vi "GUI_TRA_v1.0.0.vi"() -> ()   [LabVIEW 2011]
uses:
  Device Driver/TRAServer/HomingType_TypDef.ctl
  Device Driver/TRAServer/StatusTRA_TypDef.ctl
  Device Driver/shared/OnOffTypeDef.ctl
  <vilib>/Utility/file.llb/Write To Spreadsheet File (string).vi
  <vilib>/Utility/file.llb/Write To Spreadsheet File (DBL).vi
  Device Driver/TRAServer/TRAServer.lvclass
panel:
  in  "Multicolumn Listbox 2":refnum<vi>
  in  "Main Tap 2":refnum<vi>
  out "all pos array":refnum<vi>[][](array[refnum])
  out "all status array":refnum<vi>[][](array[refnum])
  out "indecator ref array 2":refnum<vi>[](array[refnum])
  out "indecator ref array":refnum<vi>[](array[refnum])
  in  "time to wait (TCP) 2":i32=10
  in  "plot":bool=TRUE
  out "ratio(h)":bool
  out "fixsize":bool
  out "error (h)":bool
  out "Device Name (h)":string="StagingTRA1"
  in  "Main Tap":T1(tab)
  in  "stepSize":dbl
  in  "Status":T2=enum."DISABLE" caption="Status Y"
  in  "Up":bool
  in  "Down":bool
  in  "Right":bool
  in  "Left":bool
  in  "Status":T2=enum."DISABLE" caption="Status X"
  in  "Position":dbl=2.54999 caption="X"
  in  "Position":dbl=3.05 caption="Y"
  in  "Mirror":T3(ring)
  in  "backlash":dbl
  in  "backlash":dbl
  in  "device status":string
  in  "Home 3":bool=TRUE
  in  "Home 2":bool=TRUE
  out "Status.Axis 6":T2=enum."DISABLE" caption="Status X"
  out "Status.Axis 5":T2=enum."DISABLE" caption="Status X"
  out "Status.Axis 4":T2=enum."DISABLE" caption="Status X"
  out "Status.Axis 3":T2=enum."DISABLE" caption="Status X"
  out "Status.Axis 2":T2=enum."DISABLE" caption="Status X"
  out "Status.Axis 1":T2=enum."DISABLE" caption="Status X"
  out "Status.Axis 1":T2=enum."DISABLE" caption="Status X"
  out "Status.Axis 2":T2=enum."DISABLE" caption="Status X"
  out "Status.Axis 3":T2=enum."DISABLE" caption="Status X"
  out "Status.Axis 4":T2=enum."DISABLE" caption="Status X"
  out "Status.Axis 5":T2=enum."DISABLE" caption="Status X"
  out "Status.Axis 6":T2=enum."DISABLE" caption="Status X"
  out "Status.Axis 7":T2=enum."DISABLE" caption="Status X"
  out "Status.Axis 8":T2=enum."DISABLE" caption="Status X"
  out "Status.Axis 9":T2=enum."DISABLE" caption="Status X"
  out "Status.Axis 10":T2=enum."DISABLE" caption="Status X"
  out "Status.Axis 11":T2=enum."DISABLE" caption="Status X"
  out "Status.Axis 12":T2=enum."DISABLE" caption="Status X"
  in  "Home 1":bool=TRUE
  in  "Path":path
  in  "Save":bool
  in  "Multicolumn Listbox":i32(listbox)
  in  "Position.Axis 1":dbl=3.05 caption="X"
  in  "Position.Axis 2":dbl=3.05 caption="Y"
  in  "Position.Axis 4":dbl=3.05 caption="X"
  in  "Position.Axis 3":dbl=3.05 caption="Y"
  in  "Position.Axis 6":dbl=3.05 caption="X"
  in  "Position.Axis 5":dbl=3.05 caption="Y"
  in  "Position.Axis 18":dbl=3.05 caption="X"
  in  "Position.Axis 17":dbl=3.05 caption="Y"
  in  "Position.Axis 16":dbl=3.05 caption="X"
  in  "Position.Axis 15":dbl=3.05 caption="Y"
  in  "Position.Axis 14":dbl=3.05 caption="X"
  in  "Position.Axis 13":dbl=3.05 caption="Y"
  in  "Position.Axis 12":dbl=3.05 caption="X"
  in  "Position.Axis 11":dbl=3.05 caption="Y"
  in  "Position.Axis 10":dbl=3.05 caption="X"
  in  "Position.Axis 9":dbl=3.05 caption="Y"
  in  "Position.Axis 8":dbl=3.05 caption="Y"
  in  "Position.Axis 7":dbl=3.05 caption="X"
  in  "take images":bool
  out "appended array 4":cluster{dbl[], dbl[]}[](graph)=[{[2.61999, 2.61999, 2.61999, 2.61999, 2.61999, 2.54999, 2.54999, 2.54999, 2.61999, 2.61999, 2.61999, 2.61999, 2.61999, 2.61999, 2.61999, 2.61999, 2.54999, 2.54999, 2.54999, 2.54999, 2.61999, 2.61999, 2.61999, 2.61999, 2.54999, 2.54999, 2.54999, 2.54999, 2.54999, 2.61999, 2.61999, 2.61999, 2.61999, 2.61999, 2.54999, 2.54999, 2.54999, 2.54999, 2.54999, 2.54999, 2.61999, 2.61999, 2.61999, 2.61999, 2.61999, 2.61999, 2.54999, 2.54999, 2.54999, 2.54999, 2.61999, 2.61999, 2.61999, 2.61999, 2.61999, 2.54999, 2.54999, 2.54999, 2.54999, 2.54999, 2.54999, 2.54999, 2.61999, 2.61999, 2.61999, 2.61999, 2.54999, 2.54999, 2.54999, 2.54999, 2.54999], [996.2185404112603, 996.2460308148665, 994.1496486272678, 998.7915023053579, 996.3196323980634, 265.669555365363, 264.7882927224205, 267.27969725631124, 994.8056886268479, 992.8157487597332, 992.2169788382226, 990.0215093697223, 989.2692287534538, 988.7651210814333, 990.5036192092931, 992.6276697820945, 347.21400619272106, 346.3274754410099, 347.7159425410973, 347.6197212840648, 1080.6381556133397, 1080.9803666738012, 1077.6923028536935, 1077.2355177467846, 428.6050439635929, 431.09748494375725, 426.43735365140935, 430.62353750482026, 430.0043458296606, 1165.9498871418716, 1165.3241820611406, 1166.0434051579853, 1166.3519051620808, 1167.4644217682041, 507.5921815195333, 517.0883850300825, 513.0930897984596, 512.6890147600355, 513.2647308159968, 512.8912454994768, 1246.881151792604, 1250.3560103696768, 1245.7179280397277, 1246.9677966068903, 1241.068054061203, 1241.5155828580523, 592.335370569153, 590.9527472862601, 588.8811226154211, 589.719263974882, 1405.9747477323428, 1407.8766627783912, 1406.4952048343364, 1409.4124134566805, 1405.4464710787665, 760.1565207707026, 759.594963999964, 758.1813996603448, 759.2432653857956, 756.2278502460146, 756.5241547459909, 753.8745997695793, 1502.5556451089142, 1498.9033319136602, 1492.5979471521061, 1496.3700352185133, 834.5618585239824, 837.9834154090041, 833.3014837472118, 832.3892628186035, 832.2888350246396]}, {[3.05, 3.05, 3.05, 3.05, 3.05, 3.05, 3.05, 3.05, 3.05, 3.05, 3.05, 3.05, 3.05, 3.05, 3.05, 3.05, 3.05, 3.05, 3.05, 3.05, 3.05, 3.05, 3.05, 3.05, 3.05, 3.05, 3.05, 3.05, 3.05, 3.05, 3.05, 3.05, 3.05, 3.05, 3.05, 3.05, 3.05, 3.05, 3.05, 3.05, 3.05, 3.05, 3.05, 3.05, 3.05, 3.05, 3.05, 3.05, 3.05, 3.05, 3.05, 3.05, 3.05, 3.05, 3.05, 3.05, 3.05, 3.05, 3.05, 3.05, 3.05, 3.05, 3.05, 3.05, 3.05, 3.05, 3.05, 3.05, 3.05, 3.05, 3.05], [545.600518314844, 546.2546431856922, 545.7145718356037, 545.7515341627908, 541.8426362608479, 547.2720786977828, 549.7420699869986, 547.0156395816471, 539.5624669855288, 540.3586912538148, 540.3780469257925, 538.7175456649085, 539.4764869505301, 539.156626637365, 542.14725252277, 543.0702728367195, 546.8990332633276, 545.2257778331418, 546.39846846962, 544.3799721006725, 539.780768925735, 540.2888968769458, 541.2607929342646, 538.8094606986565, 544.123211889079, 547.258172293315, 547.2634857507938, 545.0707013052162, 548.0924490847943, 537.0641641566062, 538.8037758098571, 538.2097466133315, 537.0153487890848, 535.6204485907999, 544.8752762934379, 543.9050435863884, 547.4736938429025, 545.9044751007533, 543.5908488269814, 543.6736793642327, 538.1504821175574, 538.3179818641885, 541.9503927450613, 538.1817734495421, 540.9307145593388, 539.5846809441587, 546.607251788914, 545.9652157731126, 546.6919466060039, 548.0426058632831, 536.371597111224, 538.4605570734908, 535.9758397346352, 535.7006235512454, 539.339595824224, 544.5519794558681, 548.1026938151592, 548.2595152295291, 547.8086519022737, 543.941432419384, 544.4939964861215, 545.724947909007, 537.8299601154025, 539.418355640411, 538.7853447084009, 536.2746440903762, 543.9386511945567, 546.2299898536953, 545.8455356069305, 546.826299415205, 547.3047962900782]}]
  in  "Boolean":bool
  in  "path":path=path "I:/project/Staging/TRAMotors/temp"
  out "centerY":dbl=547.3047962900782
  out "centerX":dbl=832.2888350246396
  out "local Port":u16=65435
  in  "timeout ms (slow resp)":i32=500
  in  "reset":bool
  out "image con closed":bool
  out "image \nconnection":bool
  out "image con closed 2":bool
  out "All Devices (h)":string[](array[string])=["StagingTRA1"]
  out "Remote Host":string="192.168.11.97"
  out "port or service name":u16=65434
  out "port or service name out":u16=65400
  in  "time to wait (TCP)":i32=10
  out "error out":errorcluster
  out "connections (hidden)":variant[](array[variant])=[variant(refnum<k16> refnum), variant(refnum<k16> refnum)]
  in  "time to wait (main loop)":i32=10
  out "Data String":string="Position.Axis 1,2.549990000000\r\nStatus.Axis 1,DISABLE\r\nHomingType.Axis 1,EoR- switch only\r\nDisable.Axis 1,on\r\nDisable.Axis 2,on\r\nStatus.Axis 2,DISABLE\r\nPosition.Axis 2,3.050000000000\r\n"
  in  "Local Saving Path":path
  out "Nr.":i32
  out "error (h) 2":bool
  in  "shotnumber":i32
  out "String":string="wait>>Status.Axis 1,Status.Axis 2,Status.Axis 3,Status.Axis 4,Status.Axis 5,Status.Axis 6,Position.Axis 1,Position.Axis 2,Position.Axis 3,Position.Axis 4,Position.Axis 5,Position.Axis 6,Disable.Axis 1,Disable.Axis 2,Disable.Axis 3,Disable.Axis 4,Disable.Axis 5,Disable.Axis 6,HomingType.Axis 1,HomingType.Axis 2,HomingType.Axis 3,HomingType.Axis 4,HomingType.Axis 5,HomingType.Axis 6,Home.Axis 1,Home.Axis 2,Home.Axis 3,Home.Axis 4,Home.Axis 5,Home.Axis 6,Limits.pos.Axis 1,Limits.pos.Axis 2,Limits.pos.Axis 3,Limits.pos.Axis 4,Limits.pos.Axis 5,Limits.pos.Axis 6,Limits.neg.Axis 1,Limits.neg.Axis 2,Limits.neg.Axis 3,Limits.neg.Axis 4,Limits.neg.Axis 5,Limits.neg.Axis 6,TargetPos.Axis 1,TargetPos.Axis 2,TargetPos.Axis 3,TargetPos.Axis 4,TargetPos.Axis 5,TargetPos.Axis 6,backlash.Axis 1,backlash.Axis 2,backlash.Axis 3,backlash.Axis 4,backlash.Axis 5,backlash.Axis 6"
  in  "Limits.pos":dbl=2.54999
  in  "Home":T4=enum."on"
  in  "Disable":T4=enum."on"
  in  "HomingType":T5=enum."EoR- switch only"
  in  "Disable":T4=enum."on"
  in  "HomingType":T5=enum."EoR- switch only"
  in  "Home":T4=enum."on"
  in  "Limits.pos":dbl=2.54999
  in  "Limits.neg":dbl=2.54999
  in  "Limits.neg":dbl=2.54999
  in  "Mirror 2":T3(ring)
  out "error message":string
  out "Data Connection out":bool=TRUE
  # "Position"
  # "Chassi 1"
  # "Chassi 2"
  # "Chassi 3"
  # "X"
  # "Y"
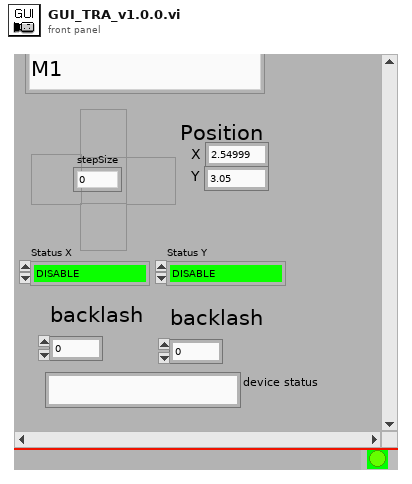
[diagram p1: front panel]
types:
  T1 = enum32{"Main", "Status", "Position", "Position 2", "Temp", "Network", "Internal", "MotorSettings"}
  T2 = typedef "TRAServer.lvclass/StatusTRA_TypDef.ctl" = enum16{"NOT REFERENCED", "CONFIGURATION", "HOMING", "MOVING", "READY", "DISABLE", "JOGGING"}
  T3 = enum16{"M1", "BS", "M3", "OAP1", "M4", "OAP2", "M5"}
  T4 = typedef "OnOffTypeDef.ctl" = enum16{"off", "on"}
  T5 = typedef "TRAServer.lvclass/HomingType_TypDef.ctl" = enum16{"MZ switch and encoder Index", "current position as HOME", "MZ switch only", "EoR- switch and encoder Index", "EoR- switch only"}
  T6 = cluster{"Chassi Nr":i32, "X":string, "Y":string, "name":string}[]
  T7 = cluster{"Chassi Nr":i32, "X":string, "Y":string, "name":string}
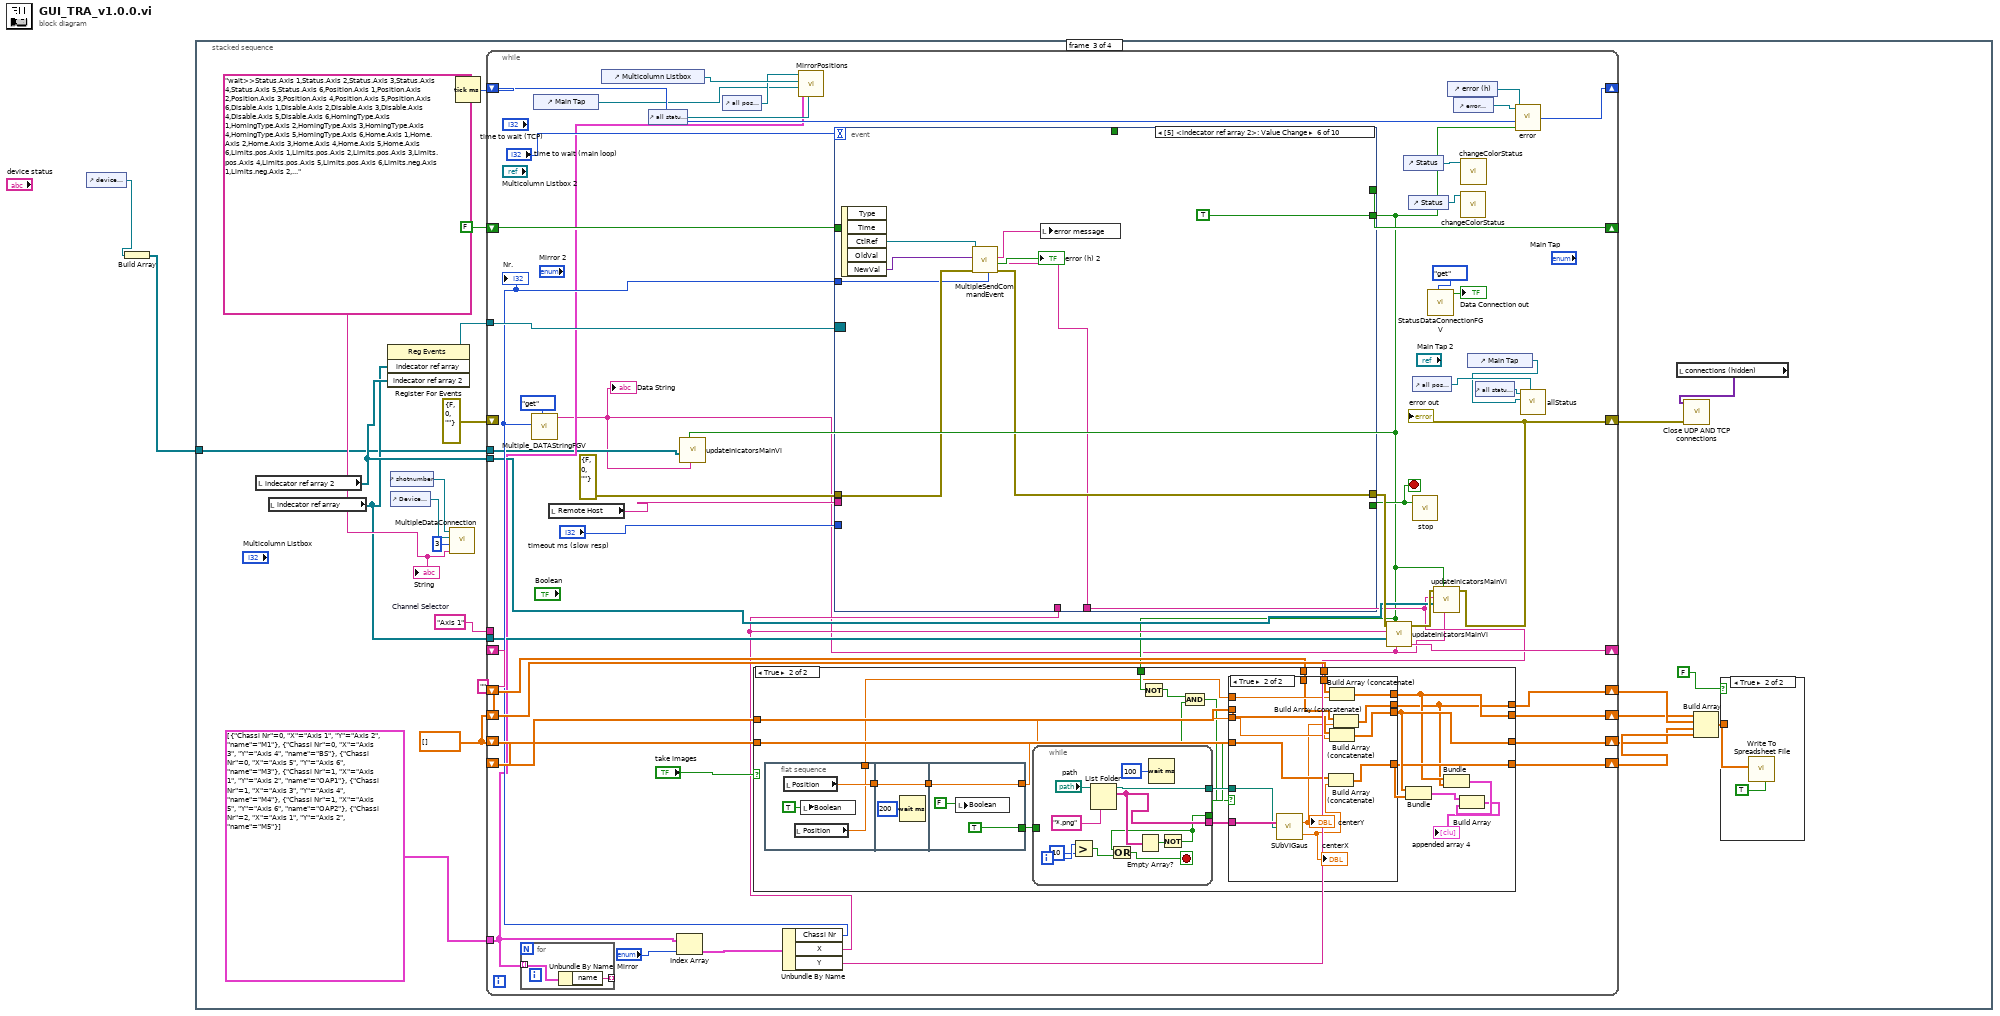
[diagram p0: block diagram]
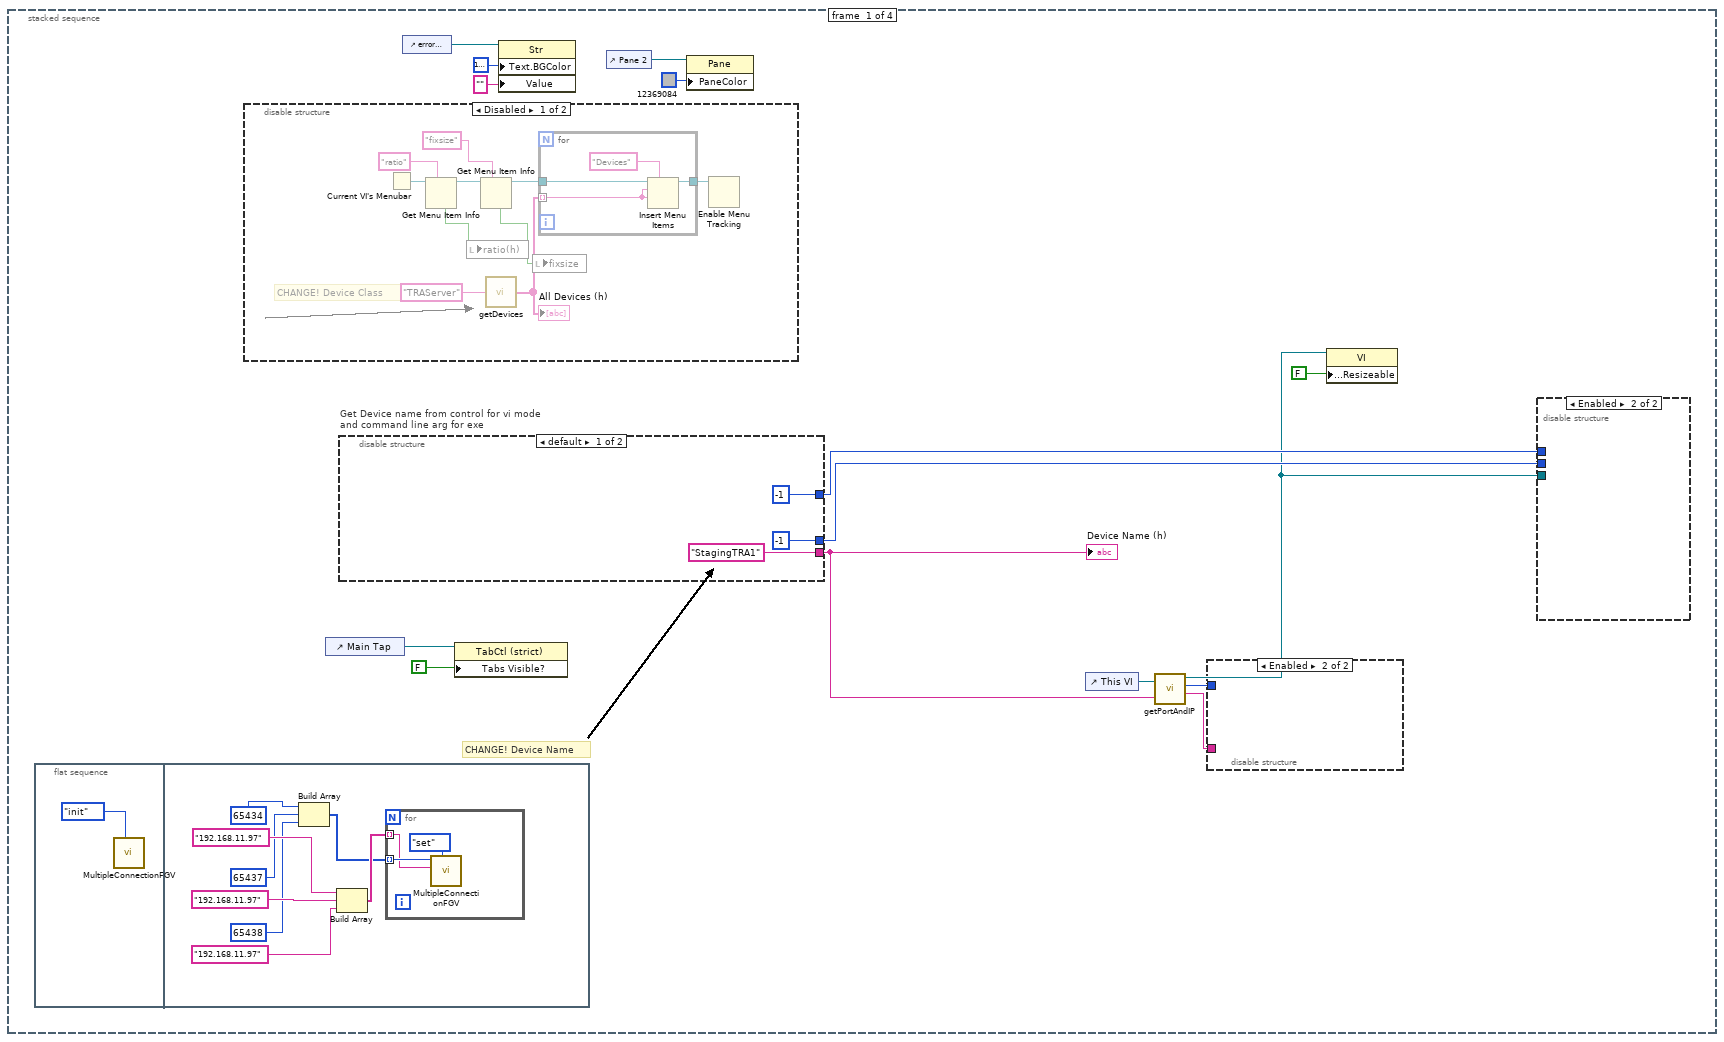
[diagram p2: hidden frame]
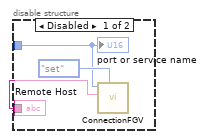
[diagram p4: hidden frame]
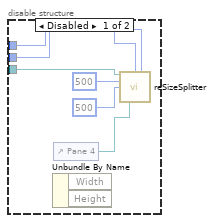
[diagram p5: hidden frame]
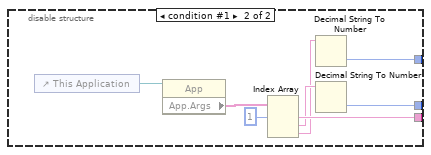
[diagram p6: hidden frame]
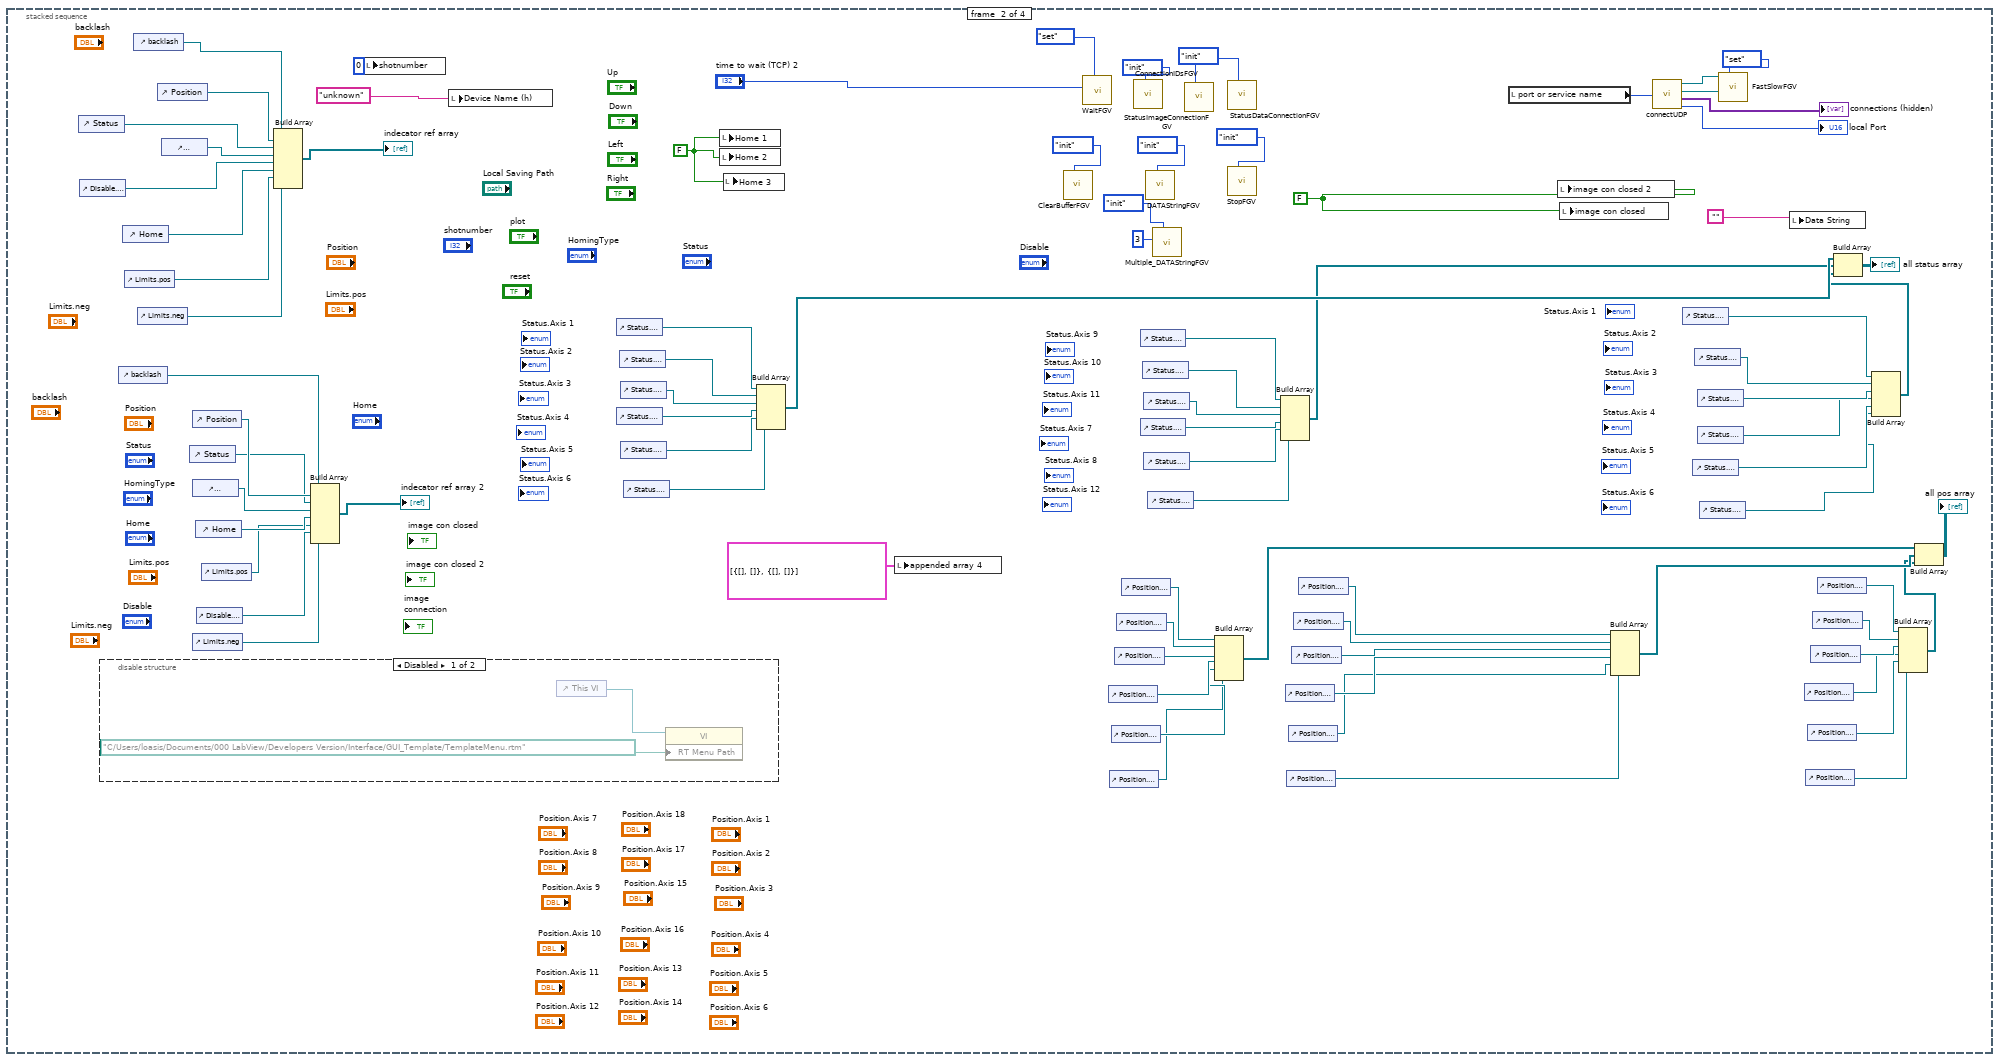
[diagram p7: hidden frame]
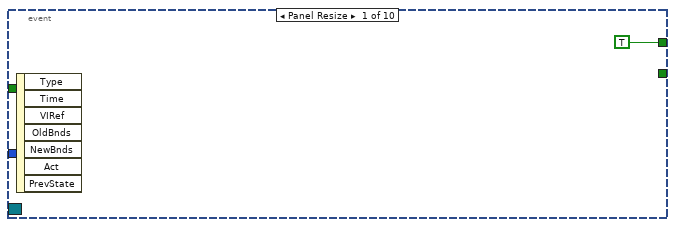
[diagram p12: hidden frame]
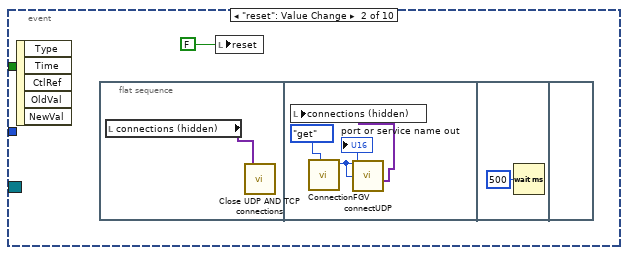
[diagram p13: hidden frame]
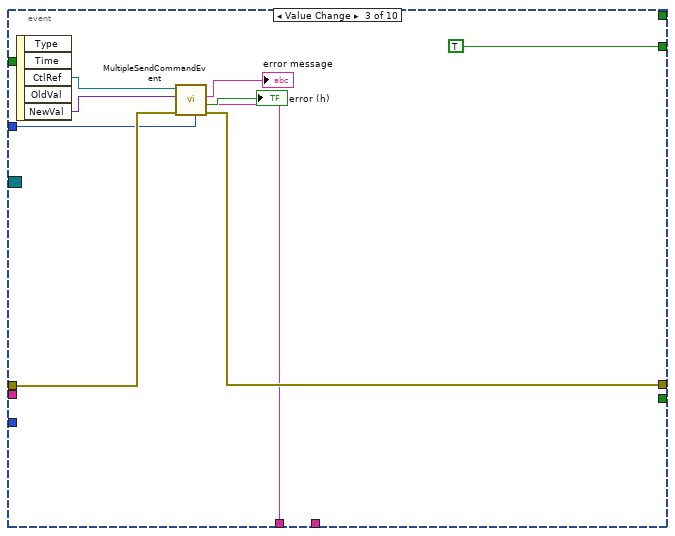
[diagram p14: hidden frame]
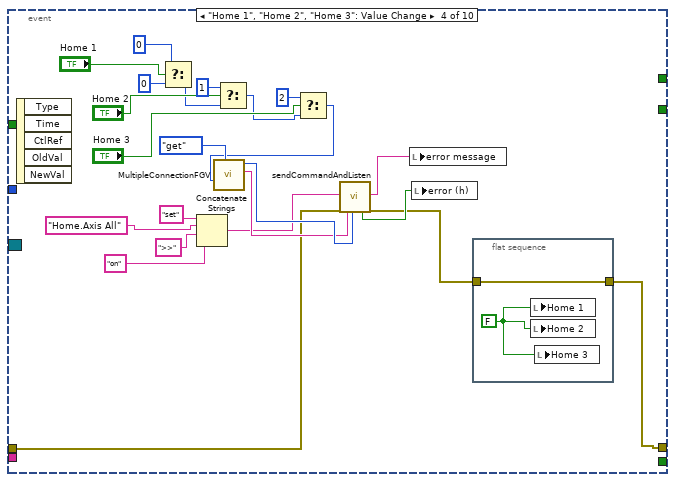
[diagram p15: hidden frame]
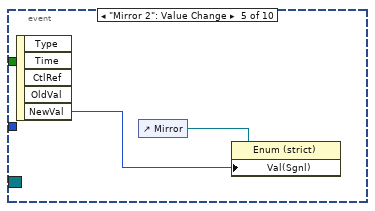
[diagram p16: hidden frame]
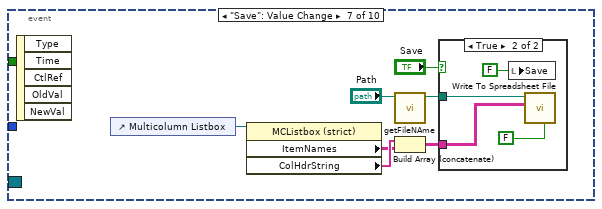
[diagram p17: hidden frame]
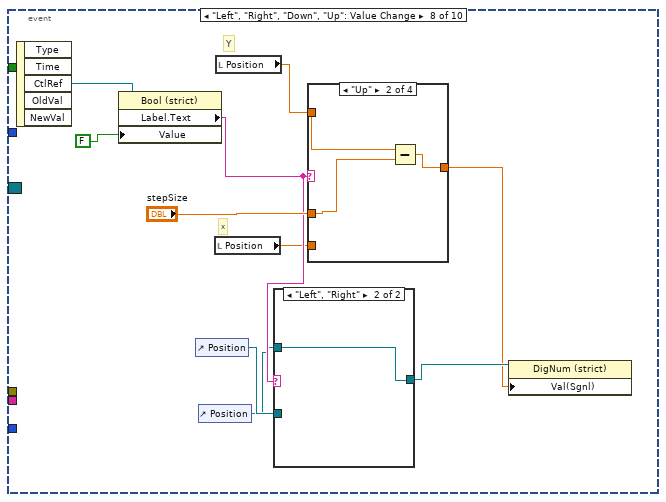
[diagram p19: hidden frame]
diagram:
  n1 = control-ref of="device status"() -> (w2:refnum<vi>)
  n2 = Build Array(w2) -> (w1:refnum<vi>[])
  n3 = stacked-sequence {
    tunnel: w1 -> [_ _ w149 _]
    frame #0 {
      # "CHANGE! Device Name"
      n4 = flat-sequence {
        frame #0 {
          n5 = call "MultipleConnectionFGV.vi"("command"=enum16{"get", "set", "init"}."init") -> ()  [unwired: 9 in, 2 out]
        }
        frame #1 {
          n6 = Build Array(u16 65434 ("port or service name"), u16 65437 ("port or service name"), u16 65438 ("port or service name")) -> (w39:u16[])
          n7 = Build Array("192.168.11.97" ("Remote Host"), "192.168.11.97" ("Remote Host"), "192.168.11.97" ("Remote Host")) -> (w40:string[])
          n8 = for {
            tunnel: w39 -> [w42] mode=indexing
            tunnel: w40 -> [w41] mode=indexing
            n9 = call "MultipleConnectionFGV.vi"("command"=enum16{"get", "set", "init"}."set", "Remote Host in"=w41, "port or service name in"=w42) -> ()  [unwired: 7 in, 2 out]
          }
        }
      }
      n10 = disable-structure shown="Disabled" {
        frame Disabled {
          # "CHANGE! Device Class"
          n11 = Current VI's Menubar() -> (w26:refnum<k9>)
          n12 = Get Menu Item Info(7:"ratio" ("item tag"), 11:w26) -> (3:w24:refnum<k9>, 4:w25:bool)  [unwired: 1 in, 5 out]
          n13 = local write "ratio(h)"(w25) -> ()
          n14 = Get Menu Item Info(7:"fixsize" ("item tag"), 11:w24) -> (3:w21:refnum<k9>, 4:w22:bool)  [unwired: 1 in, 5 out]
          n15 = call "getDevices.vi"("Device Class"="TRAServer") -> ("All Devices"=w19:string[])
          "All Devices (h)" <- w19
          n16 = local write "fixsize"(w22) -> ()
          n17 = for {
            tunnel: w21 -> [w31]
            tunnel: [w30] -> w20
            tunnel: w19 -> [w28] mode=indexing
            n18 = Insert Menu Items(5:"Devices" ("menu tag"), 7:w28, 8:w28, 9:w31) -> (3:w30:refnum<k9>)  [unwired: 2 in, 2 out]
          }
          n19 = Enable Menu Tracking(4:w20) -> ()  [unwired: 2 in, 2 out]
        }
        frame Enabled {
        }
      }
      n20 = control-ref of="Main Tap"() -> (w17:refnum<vi>)
      n21 = disable-structure "Get Device name from control for vi mode\nand command line arg for exe" shown="default" {
        disable-tunnel: ["StagingTRA1" ("Device Name for vi mode") w60] -> w13
        disable-tunnel: [i16 -1 ("left") w57] -> w15
        disable-tunnel: [i16 -1 ("left") w56] -> w14
        frame condition #0 (active) {
        }
        frame condition #1 {
          n22 = control-ref of="This Application"() -> (w63:refnum<vi>)
          n23 = property class="App"(reference=w63) -> ("App.Args"=w62:string[])  [unwired: 1 in, 2 out]
          n24 = Index Array(array=w62, index #1=1 ("index")) -> (element #1=w60:string, element #2=w59:string, element #3=w58:string)  [unwired: 2 in]
          n25 = Decimal String To Number(string=w58) -> (number=w56:i32)  [unwired: 2 in, 1 out]
          n26 = Decimal String To Number(string=w59) -> (number=w57:i32)  [unwired: 2 in, 1 out]
        }
      }
      "Device Name (h)" <- w13
      n27 = control-ref of="error message"() -> (w6:refnum<vi>)
      n28 = property class="TabCtl (strict)"(reference=w17, "Tabs Visible?"=FALSE) -> ()  [unwired: 1 in, 2 out]
      n29 = property class="Str"(reference=w6, "Text.BGColor"=u32 16777238, "Value"="") -> ()  [unwired: 1 in, 2 out]
      n30 = control-ref of="Pane 2"() -> (w4:refnum<vi>)
      n31 = property class="Pane"(reference=w4, "PaneColor"=u32 12369084) -> ()  [unwired: 1 in, 2 out]
      n32 = control-ref of="This VI"() -> (w12:refnum<vi>)
      n33 = call "getPortAndIP.vi"("This Vi"=w12, "Device Name"=w13) -> ("reference out"=w10:refnum<vi>, "port or service name"=w8:u16, "Remote Host"=w9:string)  [unwired: 1 in]
      n34 = disable-structure shown="Enabled" {
        disable-tunnel: w9 -> [w45 _]
        disable-tunnel: w8 -> [w44 _]
        frame Disabled {
          n35 = call "ConnectionFGV.vi"("command"=enum16{"get", "set", "init"}."set", "Remote Host in"=w45, "port or service name in"=w44) -> ()  [unwired: 7 in, 2 out]
          "port or service name" <- w44
          "Remote Host" <- w45
        }
        frame Enabled {
        }
      }
      n36 = property class="VI"(reference=w10, "Front Panel.Resizeable"=FALSE ("Front Panel Window:Resizable")) -> ()  [unwired: 1 in, 2 out]
      n37 = disable-structure shown="Enabled" {
        disable-tunnel: w15 -> [w52 _]
        disable-tunnel: w14 -> [w51 _]
        disable-tunnel: w10 -> [w49 _]
        frame Disabled {
          n38 = Unbundle By Name() -> ()  [unwired: 1 in, 2 out]
          n39 = control-ref of="Pane 4"() -> (w50:refnum<vi>)
          n40 = call "reSizeSplitter.vi"("this vi"=w49, "left"=w52, "top"=w51, "Width"=u32 500, "Height"=u32 500, "pane2"=w50) -> ()  [unwired: 9 in, 1 out]
        }
        frame Enabled {
        }
      }
    }
    frame #1 {
      w89 = FALSE
      w138 = enum16{"get", "set", "init"}."init" ("Command")
      w144 = FALSE ("new Device Data")
      n41 = control-ref of="Status"() -> (w127:refnum<vi>)
      n42 = control-ref of="Disable.Axis 1"() -> (w125:refnum<vi>)
      n43 = disable-structure shown="Disabled" {
        frame Disabled {
          n44 = control-ref of="This VI"() -> (w148:refnum<vi>)
          n45 = property class="VI"(reference=w148, "RT Menu Path"=path "C:/Users/loasis/Documents/000 LabView/Developers Version/Interface/GUI_Template/TemplateMenu.rtm" ("Run-Time Menu Path")) -> ()  [unwired: 1 in, 2 out]
        }
        frame Enabled {
        }
      }
      n46 = control-ref of="backlash"() -> (w65:refnum<vi>)
      n47 = control-ref of="Home"() -> (w124:refnum<vi>)
      n48 = control-ref of="Limits.pos"() -> (w123:refnum<vi>)
      n49 = control-ref of="backlash"() -> (w64:refnum<vi>)
      n50 = control-ref of="Limits.neg"() -> (w113:refnum<vi>)
      n51 = control-ref of="Position"() -> (w128:refnum<vi>)
      n52 = control-ref of="HomingType.Axis 1"() -> (w126:refnum<vi>)
      n53 = control-ref of="Status"() -> (w119:refnum<vi>)
      n54 = control-ref of="Position"() -> (w120:refnum<vi>)
      n55 = control-ref of="HomingType"() -> (w118:refnum<vi>)
      n56 = control-ref of="Limits.neg"() -> (w112:refnum<vi>)
      n57 = control-ref of="Home"() -> (w117:refnum<vi>)
      n58 = control-ref of="Disable.Axis"() -> (w115:refnum<vi>)
      n59 = control-ref of="Limits.pos"() -> (w116:refnum<vi>)
      n60 = Build Array(w64, w128, w127, w126, w125, w124, w123, w113) -> (→"indecator ref array":refnum<vi>[])
      n61 = Build Array(w65, w120, w119, w118, w117, w116, w115, w112) -> (→"indecator ref array 2":refnum<vi>[])
      n62 = local write "shotnumber"(0 ("shotnumber")) -> ()
      n63 = local write "Device Name (h)"("unknown" ("Device Name")) -> ()
      n64 = control-ref of="Status.Axis 1"() -> (w94:refnum<vi>)
      n65 = control-ref of="Status.Axis 4"() -> (w97:refnum<vi>)
      n66 = control-ref of="Status.Axis 2"() -> (w95:refnum<vi>)
      n67 = control-ref of="Status.Axis 3"() -> (w96:refnum<vi>)
      n68 = control-ref of="Status.Axis 5"() -> (w98:refnum<vi>)
      n69 = control-ref of="Status.Axis 6"() -> (w99:refnum<vi>)
      n70 = local write "Home 1"(w89) -> ()
      n71 = local write "Home 2"(w89) -> ()
      n72 = local write "Home 3"(w89) -> ()
      n73 = Build Array(w94, w95, w96, w97, w98, w99) -> (w93:refnum<vi>[])
      n74 = local write "appended array 4"(cluster{dbl[], dbl[]}[] [{[], []}, {[], []}] ("appended array 4")) -> ()
      n75 = call "ClearBufferFGV.vi"("Command"=enum16{"set", "get", "init"}."init") -> ()  [unwired: 10 in, 1 out]
      n76 = call "WaitFGV.vi"("Command"=enum16{"get", "set", "init"}."set", "milliseconds to wait"="time to wait (TCP) 2") -> ()  [unwired: 9 in, 1 out]
      n77 = control-ref of="Position.Axis 10"() -> (w85:refnum<vi>)
      n78 = control-ref of="Position.Axis 12"() -> (w83:refnum<vi>)
      n79 = control-ref of="Position.Axis 11"() -> (w84:refnum<vi>)
      n80 = control-ref of="Position.Axis 9"() -> (w86:refnum<vi>)
      n81 = control-ref of="Position.Axis 8"() -> (w87:refnum<vi>)
      n82 = control-ref of="Position.Axis 7"() -> (w88:refnum<vi>)
      n83 = call "ConnectionIDsFGV.vi"("Command"=enum16{"add", "get", "init"}."init") -> ()  [unwired: 10 in, 1 out]
      n84 = control-ref of="Status.Axis 9"() -> (w105:refnum<vi>)
      n85 = control-ref of="Status.Axis 7"() -> (w102:refnum<vi>)
      n86 = control-ref of="Status.Axis 10"() -> (w104:refnum<vi>)
      n87 = control-ref of="Status.Axis 11"() -> (w103:refnum<vi>)
      n88 = control-ref of="Status.Axis 8"() -> (w101:refnum<vi>)
      n89 = call "DATAStringFGV.vi"("Command"=enum16{"get", "set", "init"}."init") -> ()  [unwired: 10 in, 1 out]
      n90 = control-ref of="Status.Axis 12"() -> (w100:refnum<vi>)
      n91 = call "Multiple_DATAStringFGV.vi"("Command"=enum16{"get", "set", "init"}."init", "Nr."=3) -> ()  [unwired: 9 in, 1 out]
      n92 = call "StatusImageConnectionFGV.vi"("Command"=w138) -> ()  [unwired: 10 in, 1 out]
      n93 = Build Array(w88, w87, w86, w85, w84, w83) -> (w70:refnum<vi>[])
      n94 = call "StatusDataConnectionFGV.vi"("Command"=w138) -> ()  [unwired: 10 in, 1 out]
      n95 = call "StopFGV.vi"("Command"=enum16{"set", "get", "init"}."init") -> ()  [unwired: 10 in, 1 out]
      n96 = Build Array(w105, w104, w103, w102, w101, w100) -> (w92:refnum<vi>[])
      n97 = control-ref of="Position.Axis 16"() -> (w79:refnum<vi>)
      n98 = control-ref of="Position.Axis 14"() -> (w77:refnum<vi>)
      n99 = control-ref of="Position.Axis 13"() -> (w78:refnum<vi>)
      n100 = control-ref of="Position.Axis 15"() -> (w80:refnum<vi>)
      n101 = control-ref of="Position.Axis 17"() -> (w81:refnum<vi>)
      n102 = control-ref of="Position.Axis 18"() -> (w82:refnum<vi>)
      n103 = local read "port or service name"() -> (w134:u16)
      n104 = local write "image con closed 2"(w144) -> ()
      n105 = local write "image con closed"(w144) -> ()
      n106 = Build Array(w82, w81, w80, w79, w78, w77) -> (w69:refnum<vi>[])
      n107 = call "connectUDP.vi"("port or service name"=w134) -> ("fast ID (h)"=w133:refnum<k16>, "slow ID (h)"=w132:refnum<k16>, "connections (hidden)"=→"connections (hidden)":variant[], "local Port"=→"local Port":u16)
      n108 = control-ref of="Status.Axis 1"() -> (w111:refnum<vi>)
      n109 = control-ref of="Status.Axis 5"() -> (w107:refnum<vi>)
      n110 = control-ref of="Status.Axis 2"() -> (w110:refnum<vi>)
      n111 = control-ref of="Status.Axis 3"() -> (w109:refnum<vi>)
      n112 = control-ref of="Status.Axis 4"() -> (w108:refnum<vi>)
      n113 = control-ref of="Status.Axis 6"() -> (w106:refnum<vi>)
      n114 = call "FastSlowFGV.vi"("Command"=enum16{"get", "set", "init"}."set", "slow ID"=w132, "fast ID"=w133) -> ()  [unwired: 7 in, 2 out]
      n115 = local write "Data String"("") -> ()
      n116 = control-ref of="Position.Axis 4"() -> (w73:refnum<vi>)
      n117 = control-ref of="Position.Axis 6"() -> (w71:refnum<vi>)
      n118 = control-ref of="Position.Axis 5"() -> (w72:refnum<vi>)
      n119 = control-ref of="Position.Axis 3"() -> (w74:refnum<vi>)
      n120 = control-ref of="Position.Axis 2"() -> (w75:refnum<vi>)
      n121 = control-ref of="Position.Axis 1"() -> (w76:refnum<vi>)
      n122 = Build Array(w111, w110, w109, w108, w107, w106) -> (w91:refnum<vi>[])
      n123 = Build Array(w93, w92, w91) -> (→"all status array":refnum<vi>[][])
      n124 = Build Array(w76, w75, w74, w73, w72, w71) -> (w68:refnum<vi>[])
      n125 = Build Array(w70, w69, w68) -> (→"all pos array":refnum<vi>[][])
    }
    frame #2 {
      w154 = "wait>>Status.Axis 1,Status.Axis 2,Status.Axis 3,Status.Axis 4,Status.Axis 5,Status.Axis 6,Position.Axis 1,Position.Axis 2,Position.Axis 3,Position.Axis 4,Position.Axis 5,Position.Axis 6,Disable.Axis 1,Disable.Axis 2,Disable.Axis 3,Disable.Axis 4,Disable.Axis 5,Disable.Axis 6,HomingType.Axis 1,HomingType.Axis 2,HomingType.Axis 3,HomingType.Axis 4,HomingType.Axis 5,HomingType.Axis 6,Home.Axis 1,Home.Axis 2,Home.Axis 3,Home.Axis 4,Home.Axis 5,Home.Axis 6,Limits.pos.Axis 1,Limits.pos.Axis 2,Limits.pos.Axis 3,Limits.pos.Axis 4,Limits.pos.Axis 5,Limits.pos.Axis 6,Limits.neg.Axis 1,Limits.neg.Axis 2,Limits.neg.Axis 3,Limits.neg.Axis 4,Limits.neg.Axis 5,Limits.neg.Axis 6,TargetPos.Axis 1,TargetPos.Axis 2,TargetPos.Axis 3,TargetPos.Axis 4,TargetPos.Axis 5,TargetPos.Axis 6,backlash.Axis 1,backlash.Axis 2,backlash.Axis 3,backlash.Axis 4,backlash.Axis 5,backlash.Axis 6,device status" ("String")
      w161 = dbl[] []
      w162 = "Axis 1"  # Channel Selector
      n126 = local read "indecator ref array 2"() -> (w153:refnum<vi>[])
      n127 = local read "indecator ref array"() -> (w152:refnum<vi>[])
      n128 = register-events(w152, w153) -> (reference out=w163:refnum<event-registration>)  [unwired: 2 in, 1 out]
      n129 = control-ref of="shotnumber"() -> (w165:refnum<vi>)
      n130 = control-ref of="Device Name (h)"() -> (w164:refnum<vi>)
      n131 = call "MultipleDataConnection.vi"("Subscriber list 2"=w154, "Nr."=3, "Device Name (h)"=w164, "shotnumber"=w165) -> ()
      n132 = Tick Count (ms)() -> (millisecond timer value=w167:u32)
      n133 = while {
        shift-right: [w195] -> w170
        shift-left: errorcluster {"status"=FALSE, "code"=0, "source"=""} ("error out") -> [_]
        tunnel: w152 -> [w193]
        shift-right: [w216] -> _
        shift-left: FALSE -> [w217]
        shift-right: [w215] -> _
        shift-left: w167 -> [w214]
        shift-right: [w209] -> _
        shift-left: "" ("Data String") -> [_]
        tunnel: w163 -> [w211]
        tunnel: w162 -> [_]
        shift-right: [w204] -> w158
        shift-left: w161 -> [w206]
        shift-right: [w203] -> w159
        shift-left: w161 -> [w205]
        shift-right: [w199] -> w157
        shift-left: w161 -> [w198]
        shift-right: [w201] -> w156
        shift-left: w161 -> [w200]
        tunnel: w153 -> [w192]
        tunnel: T6 [{"Chassi Nr"=0, "X"="Axis 1", "Y"="Axis 2", "name"="M1"}, {"Chassi Nr"=0, "X"="Axis 3", "Y"="Axis 4", "name"="BS"}, {"Chassi Nr"=0, "X"="Axis 5", "Y"="Axis 6", "name"="M3"}, {"Chassi Nr"=1, "X"="Axis 1", "Y"="Axis 2", "name"="OAP1"}, {"Chassi Nr"=1, "X"="Axis 3", "Y"="Axis 4", "name"="M4"}, {"Chassi Nr"=1, "X"="Axis 5", "Y"="Axis 6", "name"="OAP2"}, {"Chassi Nr"=2, "X"="Axis 1", "Y"="Axis 2", "name"="M5"}] -> [w179]
        tunnel: w149 -> [w176]
        stop <- w212 stop-if-true
        n134 = for {
          tunnel: w179 -> [w223] mode=indexing
          tunnel: [w222] -> _ mode=indexing
          n135 = Unbundle By Name(w223) -> ("name"=w222:string)
        }
        n136 = control-ref of="Main Tap"() -> (w177:refnum<vi>)
        n137 = local read "Remote Host"() -> (w219:string)
        n138 = control-ref of="Multicolumn Listbox"() -> (w182:refnum<vi>)
        n139 = control-ref of="all status array"() -> (w180:refnum<vi>)
        n140 = Index Array(array=w179, index="Mirror") -> (element=w183:T7)
        n141 = control-ref of="all pos array"() -> (w181:refnum<vi>)
        n142 = Unbundle By Name(w183) -> ("Chassi Nr"=w194:i32, "X"=w191:string, "Y"=w190:string)
        "Nr." <- w194
        n143 = call "Multiple_DATAStringFGV.vi"("Command"=enum16{"get", "set", "init"}."get", "Nr."=w194) -> ("Data String out"=w174:string)  [unwired: 9 in]
        "Data String" <- w174
        n144 = call "MirrorPositions.vi"("all status array"=w180, "Array"=w179, "reference"=w177, "Multicolumn Listbox 2"=w182, "Array in"=w181) -> ()  [unwired: 7 in]
        n145 = event shown="[5] <indecator ref array 2>: Value Change" {
          selector: w211 -> [_ _ _ _ _ _ _ _ _ _]
          dyn-events: _ -> [_ _ _ _ _ _ _ _ _ _]
          timeout: "time to wait (main loop)" -> [_ _ _ _ _ _ _ _ _ _]
          tunnel: [_ _ w300 w303 _ w336 _ _ w375 w377] -> w218
          tunnel: w219 -> [_ _ _ _ _ _ _ _ _ _]
          tunnel: "timeout ms (slow resp)" -> [_ _ _ _ _ _ _ _ _ _]
          tunnel: errorcluster {"status"=FALSE, "code"=0, "source"=""} ("error out") -> [_ _ w297 w320 _ w334 _ _ w375 w378]
          tunnel: [_ _ TRUE _ _ TRUE _ _ _ _] -> w175
          tunnel: [_ _ _ _ _ _ _ _ _ w383] -> w212
          tunnel: [_ _ _ _ _ _ _ _ w374 w380] -> _
          tunnel: w217 -> [_ _ _ _ _ _ _ _ w374 _]
          tunnel: [TRUE _ _ _ _ _ _ _ _ _] -> w216
          tunnel: w194 -> [_ _ w295 _ _ w332 _ _ _ _]
          tunnel: w191 -> [_ _ w294 _ _ _ _ _ _ _]
          tunnel: w190 -> [_ _ _ _ _ w331 _ _ _ _]
          event Panel Resize {
            n146 = event-data() -> ()  [unwired: 1 in, 7 out]
          }
          event "reset": Value Change {
            n147 = event-data() -> ()  [unwired: 1 in, 5 out]
            n148 = flat-sequence {
              frame #0 {
                n149 = local read "connections (hidden)"() -> (w289:variant[])
                n150 = call "Close UDP AND TCP connections.vi"("appended array"=w289) -> ()  [unwired: 7 in]
              }
              frame #1 {
                n151 = call "ConnectionFGV.vi"("command"=enum16{"get", "set", "init"}."get") -> ("port or service name out"=w291:u16)  [unwired: 9 in, 1 out]
                "port or service name out" <- w291
                n152 = call "connectUDP.vi"("port or service name"=w291) -> ("connections (hidden)"=w290:variant[])  [unwired: 3 out]
                n153 = local write "connections (hidden)"(w290) -> ()
              }
              frame #2 {
                n154 = Wait (ms)(milliseconds to wait=u32 500) -> ()  [unwired: 1 out]
              }
              frame #3 {
              }
            }
            n155 = local write "reset"(FALSE ("reset")) -> ()
          }
          event Value Change {
            n156 = event-data() -> ("CtlRef"=w302:refnum<vi>, "NewVal"=w301:variant)  [unwired: 1 in, 3 out]
            n157 = call "MultipleSendCommandEvent.vi"("Nr."=w295, "error out 2"=w297, "Channel Selector"=w294, "NewVal"=w301, "CtlRef"=w302) -> ("error out"=w300:errorcluster, "error (h)"=→"error (h)":bool, "error message"=→"error message":string)  [unwired: 3 in, 1 out]
          }
          event "Home 1", "Home 2", "Home 3": Value Change {
            n158 = event-data() -> ()  [unwired: 1 in, 5 out]
            n159 = Select(t=0 ("Nr."), s="Home 1", f=0) -> (s? t:f=w307:i32)
            n160 = Concatenate Strings("set", "Home.Axis All" ("string"), ">>" ("string"), "on" ("string")) -> (w322:string)
            n161 = Select(t=1 ("Nr."), s="Home 2", f=w307) -> (s? t:f=w308:i32)
            n162 = Select(t=2 ("Nr."), s="Home 3", f=w308) -> (s? t:f=w305:i32)
            n163 = call "MultipleConnectionFGV.vi"("command"=enum16{"get", "set", "init"}."get", "Nr."=w305) -> ("Remote Host out"=w324:string, "port or service name out"=w325:u16)  [unwired: 8 in]
            n164 = call "sendCommandAndListen.vi"("command in"=w322, "error in"=w320, "Remote Host"=w324, "port or service name"=w325) -> ("error"=w318:bool, "error message"=w319:string, "error out"=w304:errorcluster)  [unwired: 8 in, 5 out]
            n165 = local write "error message"(w319) -> ()
            n166 = local write "error (h)"(w318) -> ()
            n167 = flat-sequence {
              tunnel: w304 -> [w327]
              tunnel: [w327] -> w303
              frame #0 {
                w326 = FALSE
                n168 = local write "Home 1"(w326) -> ()
                n169 = local write "Home 2"(w326) -> ()
                n170 = local write "Home 3"(w326) -> ()
              }
            }
          }
          event "Mirror 2": Value Change {
            n171 = event-data() -> ("NewVal"=w328:T3)  [unwired: 1 in, 4 out]
            n172 = control-ref of="Mirror"() -> (w329:refnum<vi>)
            n173 = property class="Enum (strict)"(reference=w329, "Val(Sgnl)"=w328) -> ()  [unwired: 1 in, 2 out]
          }
          event Value Change {
            n174 = event-data() -> ("CtlRef"=w338:refnum<vi>, "NewVal"=w337:variant)  [unwired: 1 in, 3 out]
            n175 = call "MultipleSendCommandEvent.vi"("Nr."=w332, "error out 2"=w334, "Channel Selector"=w331, "NewVal"=w337, "CtlRef"=w338) -> ("error out"=w336:errorcluster, "error (h)"=→"error (h) 2":bool, "error message"=w330:string)  [unwired: 3 in, 1 out]
            n176 = local write "error message"(w330) -> ()
          }
          event "Save": Value Change {
            n177 = event-data() -> ()  [unwired: 1 in, 5 out]
            n178 = control-ref of="Multicolumn Listbox"() -> (w345:refnum<vi>)
            n179 = property class="MCListbox (strict)"(reference=w345) -> ("ItemNames"=w343:string[][], "ColHdrString"=w344:string[])  [unwired: 1 in, 2 out]
            n180 = call "getFileNAme.vi"("Path"="Path") -> ("appended path"=w339:path)  [unwired: 9 in, 1 out]
            n181 = Build Array (concatenate)(w344, w343) -> (w341:string[][])
            n182 = case shown="True" "Save" {
              tunnel: w339 -> [_ w348]
              tunnel: w341 -> [_ w347]
              frame False {
              }
              frame True {
                n183 = local write "Save"(FALSE ("Save")) -> ()
                n184 = call-poly <vilib>:"Write To Spreadsheet File.vi"("transpose? (no:F)"=FALSE, "2D data"=w347, "file path (dialog if empty)"=w348) -> ()  [unwired: 5 in, 1 out]
              }
            }
          }
          event "Left", "Right", "Down", "Up": Value Change {
            # "Y"
            # "x"
            n185 = event-data() -> ("CtlRef"=w359:refnum<vi>)  [unwired: 1 in, 4 out]
            n186 = property class="Bool (strict)"(reference=w359, "Value"=FALSE) -> ("Label.Text"=w356:string)  [unwired: 1 in, 2 out]
            n187 = control-ref of="Position"() -> (w351:refnum<vi>)
            n188 = control-ref of="Position"() -> (w350:refnum<vi>)
            n189 = local read "Position"() -> (w352:dbl)
            n190 = local read "Position"() -> (w357:dbl)
            n191 = case shown="\"Left\", \"Right\"" w356 {
              tunnel: w350 -> [_ w361]
              tunnel: w351 -> [w360 _]
              tunnel: [w360 w361] -> w355
              frame "Down", "Up", Default {
              }
              frame "Left", "Right" {
              }
            }
            n192 = case shown="\"Up\"" w356 {
              tunnel: w352 -> [w363 _ _ w373]
              tunnel: "stepSize" -> [w364 w366 w369 w372]
              tunnel: [w362 w365 w368 w371] -> w354
              tunnel: w357 -> [_ w367 w370 _]
              frame "Right" {
                n193 = Add(x=w364, y=w363) -> (x+y=w362:dbl)
              }
              frame "Up" {
                n194 = Subtract(x=w367, y=w366) -> (x-y=w365:dbl)
              }
              frame "Down", Default {
                n195 = Add(x=w370, y=w369) -> (x+y=w368:dbl)
              }
              frame "Left" {
                n196 = Subtract(x=w373, y=w372) -> (x-y=w371:dbl)
              }
            }
            n197 = property class="DigNum (strict)"(reference=w355, "Val(Sgnl)"=w354) -> ()  [unwired: 1 in, 2 out]
          }
          event Timeout {
            n198 = event-data() -> ()  [unwired: 1 in, 2 out]
          }
          event Menu Selection (User) {
            n199 = event-data() -> ("MenuRef"=w379:refnum<k9>, "ItemTag"=w381:string)  [unwired: 1 in, 3 out]
            n200 = control-ref of="Main Tap"() -> (w376:refnum<vi>)
            n201 = call "ChangeMainTap.vi"("error in"=w378, "ItemTag"=w381, "reference"=w376) -> ("error out"=w382:errorcluster, "Boolean"=w383:bool)
            n202 = case shown="Error" w382 {
              selector: w382 -> [w384 _]
              tunnel: w379 -> [_ w390]
              tunnel: [_ w392] -> w380
              tunnel: w381 -> [_ w391]
              tunnel: [w384 errorcluster {"status"=FALSE, "code"=0, "source"=""} ("error IO")] -> w377
              frame No Error {
              }
              frame Error {
                n203 = local read "All Devices (h)"() -> (w385:string[])
                n204 = call "disableMenueItem.vi"("ItemTag"=w391, "All Devices (h)"=w385, "MenuRef"=w390) -> ("this is a Device(tag)"=w389:bool, "menu reference out"=w388:refnum<k9>)  [unwired: 1 in, 1 out]
                n205 = Get Menu Item Info(7:w391, 11:w390) -> (2:w394:string, 4:w395:bool)  [unwired: 1 in, 5 out]
                n206 = Not(x=w395) -> (.not. x?=w393:bool)
                n207 = case shown="Default" w391 {
                  selector: w391 -> [_ w401 _ _ _ _]
                  tunnel: w393 -> [w396 w399 w411 _ _ _]
                  tunnel: [_ _ TRUE _ _ _] -> w392
                  tunnel: w389 -> [_ w402 _ _ _ _]
                  tunnel: [w396 w400 w411 _ _ _] -> w387
                  frame "fixsize" {
                    n208 = control-ref of="This VI"() -> (w398:refnum<vi>)
                    n209 = Not(x=w396) -> (.not. x?=w397:bool)
                    n210 = property class="VI"(reference=w398, "Front Panel.Resizeable"=w397) -> ()  [unwired: 1 in, 2 out]
                    "fixsize" <- w396
                  }
                  frame Default {
                    n211 = case shown="True" w402 {
                      tunnel: w401 -> [_ w410]
                      tunnel: [_ w406] -> w400
                      tunnel: w399 -> [_ w406]
                      frame False {
                      }
                      frame True {
                        n212 = control-ref of="reset"() -> (w408:refnum<vi>)
                        n213 = control-ref of="This VI"() -> (w409:refnum<vi>)
                        n214 = call "getPortAndIP.vi"("This Vi"=w409, "Device Name"=w410) -> ("port or service name"=w404:u16, "Remote Host"=w405:string)  [unwired: 1 in, 1 out]
                        n215 = local write "port or service name"(w404) -> ()
                        n216 = local write "Remote Host"(w405) -> ()
                        n217 = property class="Bool (strict)"(reference=w408, "Val(Sgnl)"=TRUE ("Value (Signaling)")) -> ()  [unwired: 1 in, 2 out]
                        n218 = call "ConnectionFGV.vi"("command"=enum16{"get", "set", "init"}."set", "Remote Host in"=w405, "port or service name in"=w404) -> ()  [unwired: 7 in, 2 out]
                      }
                    }
                  }
                  frame "ratio" {
                    "ratio(h)" <- w411
                  }
                  frame "Local Saving Path" {
                    n219 = control-ref of="Local Saving Path"() -> (w413:refnum<vi>)
                    n220 = property class="Path"(reference=w413) -> (reference out=w416:refnum<vi>, "Value"=w417:path)  [unwired: 1 in, 1 out]
                    n221 = call "changePath.vi"("Local Saving in (h)"=w417) -> ("change (h)"=w415:bool, "Local Saving out (h)"=w414:path)  [unwired: 9 in]
                    n222 = case shown="True" w415 {
                      tunnel: w416 -> [_ w419]
                      tunnel: w414 -> [_ w418]
                      frame False {
                      }
                      frame True {
                        n223 = property class="Path"(reference=w419, "Val(Sgnl)"=w418) -> ()  [unwired: 1 in, 2 out]
                      }
                    }
                  }
                  frame "reset" {
                    n224 = control-ref of="reset"() -> (w421:refnum<vi>)
                    n225 = property class="Bool (strict)"(reference=w421, "Val(Sgnl)"=TRUE ("Value (Signaling)")) -> ()  [unwired: 1 in, 2 out]
                  }
                  frame "clear" {
                    n226 = control-ref of="reset"() -> (w423:refnum<vi>)
                    n227 = property class="Bool (strict)"(reference=w423, "Val(Sgnl)"=TRUE ("Value (Signaling)")) -> ()  [unwired: 1 in, 2 out]
                  }
                }
                n228 = Set Menu Item Info(6:w387, 7:w391, 10:w394, 11:w388) -> ()  [unwired: 3 in, 2 out]
              }
            }
          }
        }
        n229 = call "updateInicatorsMainVi.vi"("Data String out"=w174, "Boolean"=w175, "Array"=w176) -> ()  [unwired: 6 in, 3 out]
        n230 = case shown="True" "take images" {
          tunnel: w206 -> [w227 w244]
          tunnel: w205 -> [w226 w243]
          tunnel: [w227 w242] -> w204
          tunnel: [w226 w241] -> w203
          tunnel: w175 -> [_ w237]
          tunnel: [w225 w232] -> w201
          tunnel: w200 -> [w225 w234]
          tunnel: [w224 w231] -> w199
          tunnel: w198 -> [w224 w233]
          frame False {
          }
          frame True {
            n231 = flat-sequence {
              tunnel: [w280] -> w249
              tunnel: [w279] -> w235
              tunnel: [w282] -> w248
              tunnel: w249 -> [w282]
              tunnel: [TRUE] -> w245
              tunnel: [w284] -> w240
              tunnel: w248 -> [w284]
              frame #0 {
                n232 = local read "Position"() -> (w280:dbl)
                n233 = local read "Position"() -> (w279:dbl)
                n234 = local write "Boolean"(TRUE ("Boolean")) -> ()
              }
              frame #1 {
                n235 = Wait (ms)(milliseconds to wait=u32 200) -> ()  [unwired: 1 out]
              }
              frame #2 {
                n236 = local write "Boolean"(FALSE ("Boolean")) -> ()
              }
            }
            n237 = while {
              tunnel: [w271] -> w247
              tunnel: [w270] -> w246
              tunnel: w245 -> [_]
              tunnel: [w268] -> w239
              i -> [w274]
              stop <- w275 stop-if-true
              n238 = Greater?(x=w274, y=10) -> (0:w269:bool)
              n239 = List Folder(path="path", pattern="*.png") -> (path out=w270:path, filenames=w271:string[])  [unwired: 2 in, 2 out]
              n240 = Empty Array?(array=w271) -> (empty?=w276:bool)
              n241 = Wait (ms)(milliseconds to wait=u32 100) -> ()  [unwired: 1 out]
              n242 = Not(x=w276) -> (.not. x?=w268:bool)
              n243 = Or(x=w268, y=w269) -> (x .or. y?=w275:bool)
            }
            n244 = Not(x=w237) -> (.not. x?=w238:bool)
            n245 = And(x=w238, y=w239) -> (x .and. y?=w236:bool)
            n246 = case shown="True" w236 {
              tunnel: w247 -> [_ w267]
              tunnel: w246 -> [_ w266]
              tunnel: [w252 w265] -> w242
              tunnel: w244 -> [w252 w264]
              tunnel: [w253 w263] -> w241
              tunnel: w243 -> [w253 w262]
              tunnel: w240 -> [_ w260]
              tunnel: w235 -> [_ w259]
              tunnel: [w250 w257] -> w232
              tunnel: w234 -> [w250 w258]
              tunnel: [w251 w255] -> w231
              tunnel: w233 -> [w251 w254]
              frame False {
              }
              frame True {
                n247 = call "SUbVIGaus.vi"("filenames"=w267, "path out"=w266) -> ("centerX"=w256:dbl, "centerY"=w261:dbl)  [unwired: 5 in, 7 out]
                "centerY" <- w256
                "centerX" <- w261
                n248 = Build Array (concatenate)(w262, w261) -> (w263:dbl[])
                n249 = Build Array (concatenate)(w258, w259) -> (w257:dbl[])
                n250 = Build Array (concatenate)(w264, w260) -> (w265:dbl[])
                n251 = Build Array (concatenate)(w254, w256) -> (w255:dbl[])
              }
            }
            n252 = Bundle(w242, w241) -> (w230:cluster{dbl[], dbl[]})  [unwired: 1 in]
            n253 = Bundle(w232, w231) -> (w229:cluster{dbl[], dbl[]})  [unwired: 1 in]
            n254 = Build Array(w230, w229) -> (→"appended array 4":cluster{dbl[], dbl[]}[])
          }
        }
        n255 = call "updateInicatorsMainVi.vi"("Data String out"=w174, "Boolean"=w175, "Array"=w193, "Channel Selector"=w191, "error in"=w218) -> ("Data String out 2"=w209:string, "error out"=w196:errorcluster)  [unwired: 4 in, 1 out]
        n256 = control-ref of="Status"() -> (w189:refnum<vi>)
        n257 = control-ref of="Status"() -> (w188:refnum<vi>)
        n258 = control-ref of="all pos array"() -> (w184:refnum<vi>)
        n259 = call "stop.vi"("Boolean"=w212) -> ()
        n260 = call "StatusDataConnectionFGV.vi"("Command"=enum16{"get", "set", "init"}."get") -> ("Data Connection out"=→"Data Connection out":bool)  [unwired: 10 in]
        n261 = call "updateInicatorsMainVi.vi"("Data String out"=w174, "Boolean"=w175, "Array"=w192, "Channel Selector"=w190, "error in"=w196) -> ("error out"=w195:errorcluster)  [unwired: 4 in, 2 out]
        "error out" <- w195
        n262 = control-ref of="error (h)"() -> (w207:refnum<vi>)
        n263 = control-ref of="error message"() -> (w208:refnum<vi>)
        n264 = call "changeColorStatus.vi"("Enum in"=w188) -> ()  [unwired: 11 in]
        n265 = call "changeColorStatus.vi"("Enum in"=w189) -> ()  [unwired: 11 in]
        n266 = control-ref of="Main Tap"() -> (w178:refnum<vi>)
        n267 = control-ref of="all status array"() -> (w185:refnum<vi>)
        n268 = call "error.vi"("Boolean"=w175, "millisecond timer value"=w214, "reference"=w207, "error message"=w208) -> ("millisecond timer value 2"=w215:u32)
        n269 = call "allStatus.vi"("all pos array 2"=w184, "generic class reference"=w178, "Array in"=w185) -> ()  [unwired: 9 in]
      }
      n270 = local read "connections (hidden)"() -> (w169:variant[])
      n271 = call "Close UDP AND TCP connections.vi"("error in"=w170, "appended array"=w169) -> ()  [unwired: 6 in]
      n272 = Build Array(w156, w157, w158, w159) -> (w160:dbl[][])
      n273 = case shown="True" FALSE {
        tunnel: w160 -> [_ w173]
        frame False {
        }
        frame True {
          n274 = call-poly <vilib>:"Write To Spreadsheet File.vi"("transpose? (no:F)"=TRUE, "2D data"=w173) -> ()  [unwired: 6 in, 1 out]
        }
      }
      "String" <- w154
    }
    frame #3 {
      n275 = control-ref of="Main  Control"() -> (w425:refnum<vi>)
      n276 = property class="TabCtl (strict)"(reference=w425, "Tabs Visible?"=TRUE) -> ()  [unwired: 1 in, 2 out]
      n277 = property class="TabCtl (strict)"(reference=w425, "Tab Location"=enum32{"Top", "Bottom", "Left", "Right"}."Bottom") -> ()  [unwired: 1 in, 2 out]
      n278 = flat-sequence {
        frame #0 {
          n279 = Wait (ms)(milliseconds to wait=u32 0) -> ()  [unwired: 1 out]
        }
        frame #1 {
        }
        frame #2 {
          n280 = control-ref of="This VI"() -> (w430:refnum<vi>)
          n281 = case shown="True" FALSE {
            tunnel: w430 -> [w431 w434]
            tunnel: [w431 w432] -> w429
            frame False {
            }
            frame True {
              n282 = property class="VI" props=["Front Panel.Open"](reference=w434) -> (reference out=w433:refnum<vi>)  [unwired: 1 in, 2 out]
              n283 = invoke class="VI" method="FP.Close"(reference=w433) -> (reference out=w432:refnum<vi>)  [unwired: 2 in, 2 out]
            }
          }
          n284 = Close Reference(reference=w429) -> ()  [unwired: 1 in, 1 out]
        }
      }
    }
  }
